vi "Init.vi"(8 "error in":errorcluster, 11 "CFG Base in":refnum<class "Red-y Read Write CFG.lvclass">) -> (0 "error out":errorcluster, 3 "CFG Base out":refnum<class "Red-y Read Write CFG.lvclass">)   [LabVIEW 2023, in "Red-y Read Write CFG.lvclass"]
uses:
  Red-y Read Write CFG.lvclass
  Configuration/Configuration JSON/Configuration JSON Base/CFG JSON.lvclass/CFG JSON.ctl
  Red-y Read Write CFG.lvclass/Red-y Read Write CFG.ctl
  10b84e6e-13b1-40c4-8f9f-f4e739f15aab.vi
  <vilib>/JDP Science/JSONtext/Find Item.vi
  <vilib>/JDP Science/JSONtext/Next JSON Value.vi
  <vilib>/JDP Science/JSONtext/String Subset.vi
  <vilib>/JDP Science/JSONtext/Parsing/Advance past next JSON Value (inlined COPY).vi
  <vilib>/JDP Science/JSONtext/Parsing/Advance past whitespace.vi
  <vilib>/JDP Science/JSONtext/Parsing/Advance past String.vi
  <vilib>/JDP Science/JSONtext/Parsing/Advance past Number.vi
  <vilib>/JDP Science/JSONtext/Parsing/Advance past Line Ending.vi
  <vilib>/JDP Science/JSONtext/Parsing/Parse Full Path or Item Name.vi
  <vilib>/JDP Science/JSONtext/Parsing/Advance past Array.vi
  <vilib>/JDP Science/JSONtext/Parsing/Advance past Object.vi
  <vilib>/JDP Science/JSONtext/support/Error Cluster From Code.vi
  <vilib>/JDP Science/JSONtext/Offset/Find Item Locations by Path.vi
  <vilib>/JDP Science/JSONtext/JSON text to Variant.vi
  <vilib>/Utility/error.llb/Error Cluster From Error Code.vi
  Configuration/Configuration Semaphore/CFG Semaphore.lvclass
  <vilib>/JDP Science/JSONtext/LVClass Serializer/JSONtext LVClass Serializer.lvclass
  <vilib>/ErrorRing/Error Ring.xnode
  Voegtlin_NI_SMART_Modbus_Drivers/Voegtlin_NI_SMART_Modbus_Drivers.lvlib
  Configuration/Configuration JSON/Configuration JSON Base/CFG JSON.lvclass
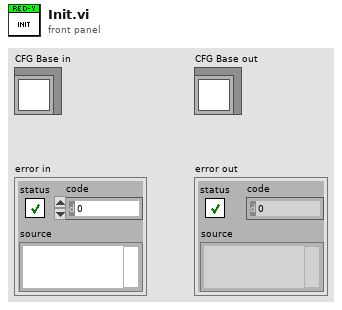
[diagram p1: front panel]
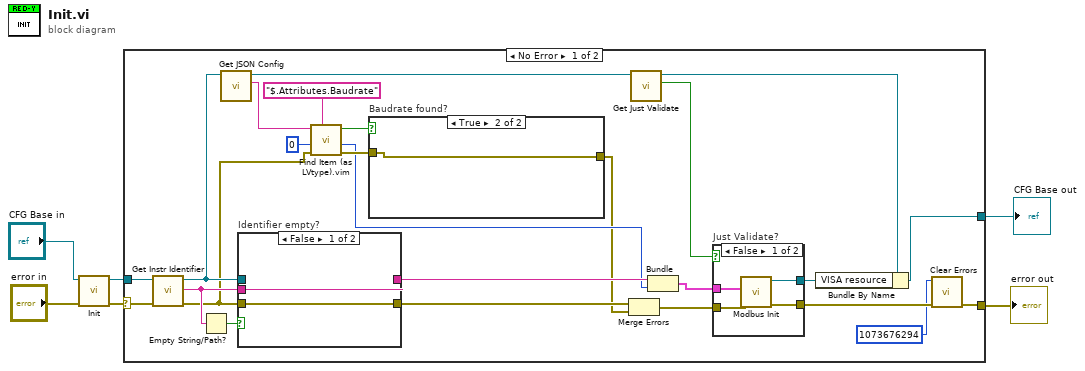
[diagram p0: block diagram]
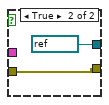
[diagram p2: hidden frame]
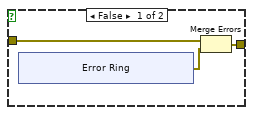
[diagram p3: hidden frame]
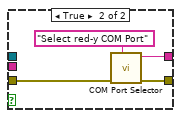
[diagram p4: hidden frame]
diagram:
  n1 = call-parent "Init.vi"("error in"="error in", "CFG Base in"="CFG Base in") -> ("error out"=w4:errorcluster, "CFG Base out"=w3:refnum<class "Red-y Read Write CFG.lvclass">)  [unwired: 8 in]
  n2 = case shown="No Error" w4 {
    selector: w4 -> [w31 w53]
    tunnel: w3 -> [w30 w54]
    tunnel: [w28 w54] -> w2
    tunnel: [w10 w53] -> w1
    frame No Error {
      n3 = call-dynamic "Get Instr Identifier.vi"("error in (no error)"=w31, "Configuration Base in"=w30) -> ("error out"=w15:errorcluster, "Instr Ident"=w27:string, "Configuration Base out"=w17:refnum<class "Red-y Read Write CFG.lvclass">)  [unwired: 7 in]
      n4 = Empty String/Path?(string/path=w27) -> (empty?=w29:bool)
      n5 = call "Get JSON Config.vi"("CFG Base in"=w17) -> ("<JSON>Config>"=w20:string, "CFG Base out"=w16:refnum<class "Red-y Read Write CFG.lvclass">)  [unwired: 9 in]
      n6 = case "Identifier empty?" shown="False" w29 {
        tunnel: w15 -> [w47 w49]
        tunnel: w27 -> [w48 _]
        tunnel: [w47 w52] -> w24
        tunnel: [w48 w50] -> w23
        tunnel: w17 -> [_ _]
        frame False {
        }
        frame True {
          n7 = call "COM Port Selector.vi"("Title"="Select red-y COM Port", "error in"=w49) -> ("error out"=w52:errorcluster, "COM Port Selected"=w50:string)  [unwired: 7 in]
        }
      }
      n8 = call "Find Item (as LVtype).vim"("$Path or Item Name"="$.Attributes.Baudrate", "error in (no error)"=w15, "Data Type and Default Value"=0, "JSON"=w20) -> ("error out"=w22:errorcluster, "Data"=w14:i32, "Found"=w21:bool)  [unwired: 4 in, 1 out]
      n9 = case "Baudrate found?" shown="True" w21 {
        tunnel: w22 -> [w39 w46]
        tunnel: [w38 w46] -> w12
        frame False {
          n10 = xnode "Error Ring"() -> ("error out"=w40:errorcluster)
          n11 = Merge Errors(w39, w40) -> (w38:errorcluster)
        }
        frame True {
        }
      }
      n12 = Merge Errors(w24, w12) -> (w13:errorcluster)
      n13 = call "Get Just Validate.vi"("CFG JSON Base in"=w16) -> ("Just Validate"=w7:bool, "CFG JSON Base out"=w8:refnum<class "Red-y Read Write CFG.lvclass">)  [unwired: 9 in]
      n14 = Bundle("COM Port Selected"=w23, "Data"=w14) -> (w11:cluster{"COM Port Selected":string, "Data":i32})  [unwired: 1 in]
      n15 = case "Just Validate?" shown="False" w7 {
        tunnel: [w35 refnum<visa-resource-name> "SIM" ("VISA resource out")] -> w26
        tunnel: [w34 w37] -> w25
        tunnel: w13 -> [w33 w37]
        tunnel: w11 -> [w32 _]
        frame False {
          n16 = call "Modbus Init.vi"("error in (no error)"=w33, "Modbus Port (Port, Baudrate)"=w32) -> ("error out"=w34:errorcluster, "VISA resource out"=w35:refnum<visa-resource-name>)  [unwired: 8 in]
        }
        frame True {
        }
      }
      n17 = Bundle By Name(cluster=w8, "VISA resource"=w26) -> (w28:refnum<class "Red-y Read Write CFG.lvclass">)
      n18 = call <vilib>:"Clear Errors.vi"("error in (no error)"=w25, "specific error code to clear (0: all)"=1073676294) -> ("error out"=w10:errorcluster)  [unwired: 4 in, 1 out]
    }
    frame Error {
    }
  }
  "error out" <- w1
  "CFG Base out" <- w2
